vi "LCM[].vi"(11 "Array":u64[](array[numeric])) -> (3 "LCM":u64)   [LabVIEW 2023, in "d8.lvlib"]
uses:
  d8.lvlib
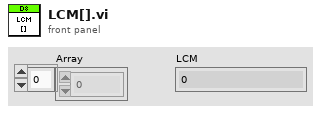
[diagram p1: front panel]
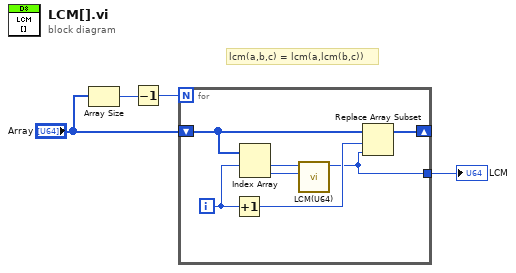
[diagram p0: block diagram]
diagram:
  # "lcm(a,b,c) = lcm(a,lcm(b,c))"
  n1 = Array Size(array="Array") -> (size(s)=w3:i32)
  n2 = Decrement(x=w3) -> (x-1=w4:i32)
  n3 = for {
    N: w4 -> [_]
    shift-right: [w8] -> _
    shift-left: "Array" -> [w9]
    tunnel: [w7] -> w2
    i -> [w11]
    n4 = Increment(x=w11) -> (x+1=w10:i32)
    n5 = Index Array(array=w9, index #1=w11) -> (element #1=w6:u64, element #2=w5:u64)  [unwired: 1 in]
    n6 = call "LCM(U64).vi"("B"=w5, "A"=w6) -> ("LCM"=w7:u64)  [unwired: 9 in]
    n7 = Replace Array Subset(array=w9, new element=w7, index=w10) -> (w8:u64[])
  }
  "LCM" <- w2
